vi "SimulateDeviceResourceUsage.vi"() -> (3 "system resources":T1 {"CPU Loads"."ISR (%)" format="%#.2f"; "CPU Loads"."Idle (%)" format="%#.2f"; "CPU Loads"."Background (%)" format="%#.2f"; "CPU Loads"."Normal (%)" format="%#.2f"; "CPU Loads"."Above Normal (%)" format="%#.2f"; "CPU Loads"."High (%)" format="%#.2g"; "CPU Loads"."Timed Structures (%)" format="%#.2g"; "CPU Loads"."Time Critical (%)" format="%#.2g"; "CPU Loads"."Total (%)" format="%#.2g"})   [LabVIEW 2017, in "SystemInfoProcess.lvlib"]
uses:
  <vilib>/addons/SystemInfoProcess/SystemInfoProcess.lvlib
  <vilib>/addons/SystemInfoProcess/controls/SystemResources.ctl
  <vilib>/addons/SystemInfoProcess/controls/Utilization.ctl
  <vilib>/addons/SystemInfoProcess/controls/CPULoad.ctl
panel:
  in  "Utilization.Memory":dbl=50.0
  in  "Utilization.CPU":dbl=50.0
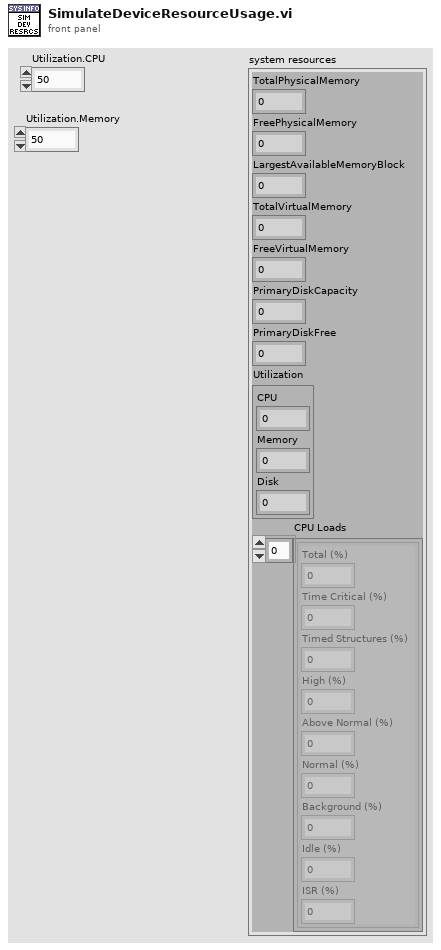
[diagram p1: front panel]
types:
  T1 = typedef "SystemInfoProcess.lvlib/SystemResources.ctl" = cluster{"TotalPhysicalMemory":dbl, "FreePhysicalMemory":dbl, "LargestAvailableMemoryBlock":dbl, "TotalVirtualMemory":dbl, "FreeVirtualMemory":dbl, "PrimaryDiskCapacity":dbl, "PrimaryDiskFree":dbl, "Utilization":T2, "CPU Loads":T3[]}
  T2 = typedef "SystemInfoProcess.lvlib/Utilization.ctl" = cluster{"CPU":dbl, "Memory":dbl, "Disk":dbl}
  T3 = typedef "SystemInfoProcess.lvlib/CPULoad.ctl" = cluster{"Total (%)":dbl, "Time Critical (%)":dbl, "Timed Structures (%)":dbl, "High (%)":dbl, "Above Normal (%)":dbl, "Normal (%)":dbl, "Background (%)":dbl, "Idle (%)":dbl, "ISR (%)":dbl}
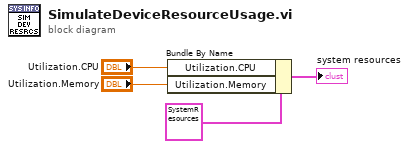
[diagram p0: block diagram]
diagram:
  n1 = Bundle By Name(cluster=T1 {"TotalPhysicalMemory"=0.0, "FreePhysicalMemory"=0.0, "LargestAvailableMemoryBlock"=0.0, "TotalVirtualMemory"=0.0, "FreeVirtualMemory"=0.0, "PrimaryDiskCapacity"=0.0, "PrimaryDiskFree"=0.0, "Utilization"={"CPU"=0.0, "Memory"=0.0, "Disk"=0.0}, "CPU Loads"=[]} ("system resources"), "Utilization.CPU"="Utilization.CPU", "Utilization.Memory"="Utilization.Memory") -> (→"system resources":T1)
